vi "data_logger_final.vi"(1 "Path":path) -> (0 "new file path (Not A Path if cancelled)":path)   [LabVIEW 2019]
uses:
  <vilib>/Utility/file.llb/Write Delimited Spreadsheet (string).vi
  <vilib>/Utility/file.llb/Write Delimited Spreadsheet (DBL).vi
panel:
  out "error out":errorcluster
  in  "error in (no error)":errorcluster
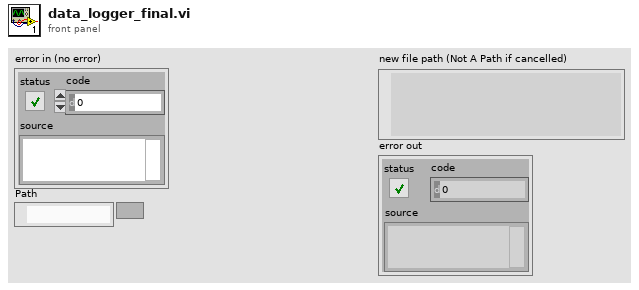
[diagram p1: front panel]
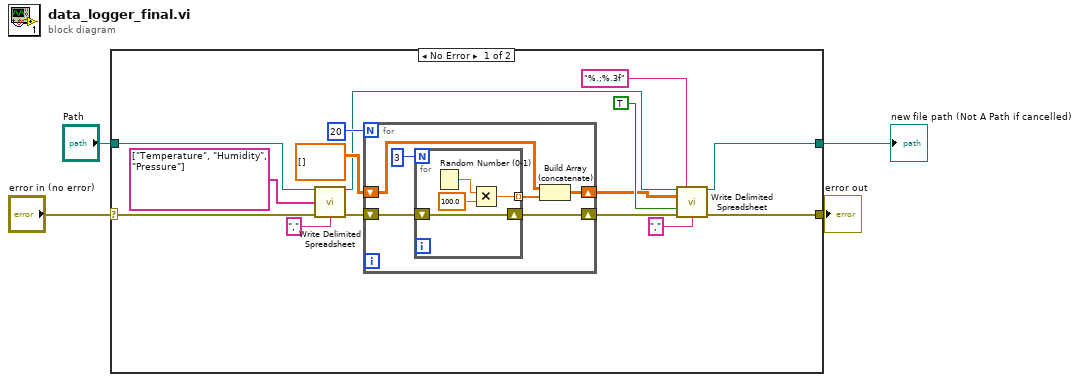
[diagram p0: block diagram]
diagram:
  n1 = case shown="No Error" "error in (no error)" {
    selector: "error in (no error)" -> [w11 w31]
    tunnel: "Path" -> [w6 w30]
    tunnel: [w14 w30] -> w4
    tunnel: [w10 w31] -> w2
    frame No Error {
      n2 = call-poly <vilib>:"Write Delimited Spreadsheet.vi"("file path (dialog if empty)"=w6, "1D data"=string[] ["Temperature", "Humidity", "Pressure"], "error in (no error)"=w11, "delimiter (\\t)"="," ("delimiter (\\t)")) -> ("new file path (Not A Path if cancelled)"=w5:path, "error out"=w9:errorcluster)  [unwired: 10 in]
      n3 = for {
        N: 20 -> [_]
        shift-right: [w20] -> w7
        shift-left: dbl[][] [] ("element") -> [w23]
        shift-right: [w21] -> w8
        shift-left: w9 -> [w22]
        n4 = for {
          N: 3 -> [_]
          tunnel: [w27] -> w24 mode=indexing
          shift-right: [w26] -> w21
          shift-left: w22 -> [w26]
          n5 = Random Number (0-1)() -> (number: 0 to 1=w29:dbl)
          n6 = Multiply(x=w29, y=100.0) -> (x*y=w27:dbl)
        }
        n7 = Build Array (concatenate)(w23, w24) -> (w20:dbl[][])
      }
      n8 = call-poly <vilib>:"Write Delimited Spreadsheet.vi"("file path (dialog if empty)"=w5, "format (%.3f)"="%.;%.3f", "2D data"=w7, "append to file? (new file:F)"=TRUE, "error in (no error)"=w8, "delimiter (\\t)"="," ("delimiter (\\t)")) -> ("new file path (Not A Path if cancelled)"=w14:path, "error out"=w10:errorcluster)  [unwired: 8 in]
    }
    frame Error {
    }
  }
  "new file path (Not A Path if cancelled)" <- w4
  "error out" <- w2
